vi "detector-exposuretime-read.vi"(2 "Loop Indicator":i32, 3 "Exposure Time (s)":sgl=1.0 caption="time target [s]") -> (0 "Progress":dbl format="%.1f%%", 1 "Elapsed Time (s)":dbl caption="elapsed time [s]" format="%.3f")   [LabVIEW 2017]
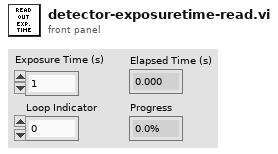
[diagram p1: front panel]
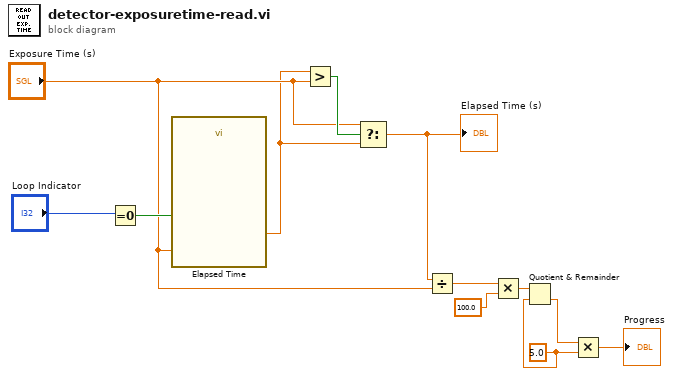
[diagram p0: block diagram]
diagram:
  w7 = 5.0 ("y")
  n1 = Equal To 0?(x="Loop Indicator") -> (x = 0?=w6:bool)
  n2 = call "Elapsed Time"("Time Target (s)"="Exposure Time (s)", "Reset"=w6) -> ("Elapsed Time (s)"=w1:dbl)  [unwired: 10 in, 7 out]
  n3 = Greater?(x=w1, y="Exposure Time (s)") -> (0:w4:bool)
  n4 = Select(t="Exposure Time (s)", s=w4, f=w1) -> (s? t:f=w2:dbl)
  "Elapsed Time (s)" <- w2
  n5 = Divide(x=w2, y="Exposure Time (s)") -> (x/y=w12:dbl)
  n6 = Multiply(x=w12, y=100.0) -> (x*y=w10:dbl)
  n7 = Quotient & Remainder(x=w10, y=w7) -> (floor(x/y)=w8:dbl)  [unwired: 1 out]
  n8 = Multiply(x=w8, y=w7) -> (x*y=→"Progress":dbl)
